vi "Get Format.vi"(8 "error in (no error)":errorcluster caption="错误输入（无错误）", 11 "SpecificString 输入":refnum<class "SpecificString.lvclass">) -> (0 "error out":errorcluster caption="错误输出", 2 "Format":string, 3 "SpecificString 输出":refnum<class "SpecificString.lvclass">)   [LabVIEW 2018, in "SpecificString.lvclass"]
uses:
  SpecificString.lvclass
  SpecificString.lvclass/SpecificString.ctl
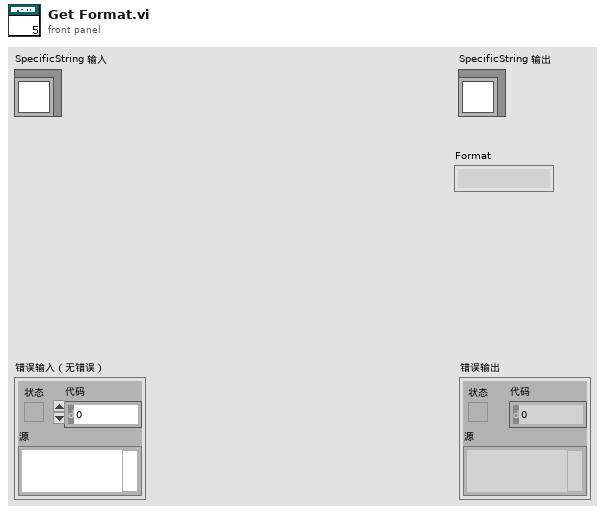
[diagram p1: front panel]
types:
  T1 = typedef "SpecificString.lvclass/State Data.ctl" = cluster{"Format":string, "Correct Color":u32, "Error Color":u32}
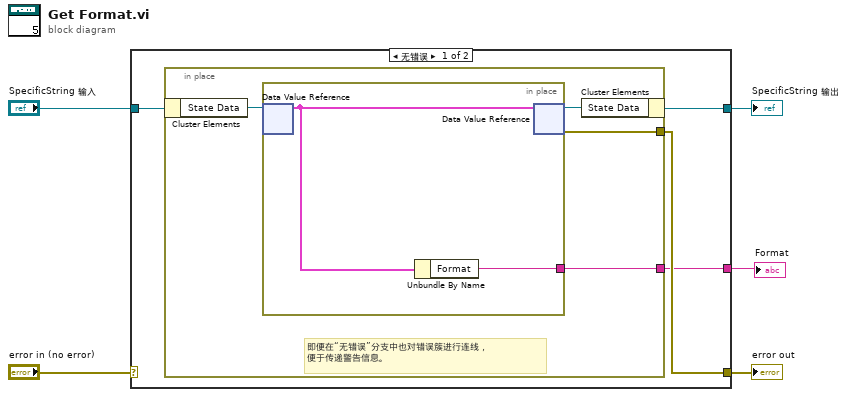
[diagram p0: block diagram]
diagram:
  n1 = case shown="无错误" "error in (no error)" {
    selector: "error in (no error)" -> [_ w17]
    tunnel: [w8 w17] -> w4
    tunnel: [w7 w16] -> w2
    tunnel: "SpecificString 输入" -> [w9 w16]
    tunnel: [w6 _] -> w1
    frame No Error {
      n2 = in-place {
        in-place-border: [w12] -> w8
        in-place-border: [w10] -> w6
        # "即便在“无错误”分支中也对错误簇进行连线，\n便于传递警告信息。"
        n3 = in-place-cluster #1(w9) -> ("State Data"=w13:refnum<data-value>)
        n4 = in-place {
          in-place-border: [w14] -> w10
          n5 = in-place-dvr #2(w13) -> (w15:T1)  [unwired: 1 out]
          n6 = Unbundle By Name(w15) -> ("Format"=w14:string)
          n7 = in-place-dvr #2(w15) -> (w11:refnum<data-value>, w12:errorcluster)
        }
        n8 = in-place-cluster #1("State Data"=w11) -> (w7:refnum<class "SpecificString.lvclass">)
      }
    }
    frame Error {
    }
  }
  "error out" <- w4
  "SpecificString 输出" <- w2
  "Format" <- w1
